vi "Get Size 1D.vi"(8 "error in (no error)":errorcluster, 11 "Abs_Array1D in":refnum<class "Abs_Array1D.lvclass">) -> (0 "error out":errorcluster, 2 "Size":i32, 3 "Abs_Array1D out":refnum<class "Abs_Array1D.lvclass">)   [LabVIEW 2021, in "Abs_Array1D.lvclass"]
uses:
  Abs_Array1D.lvclass
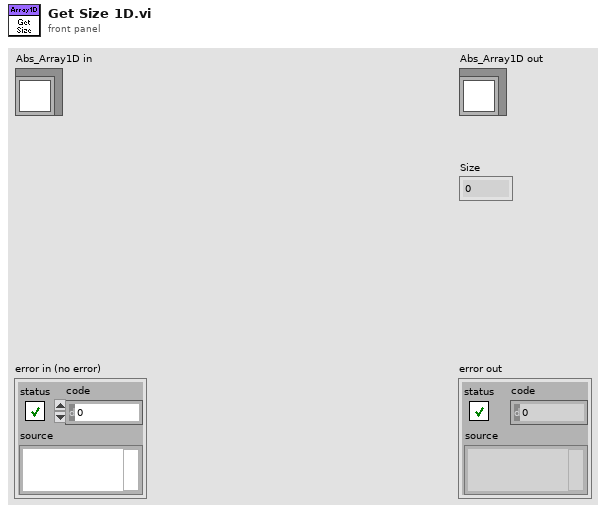
[diagram p1: front panel]
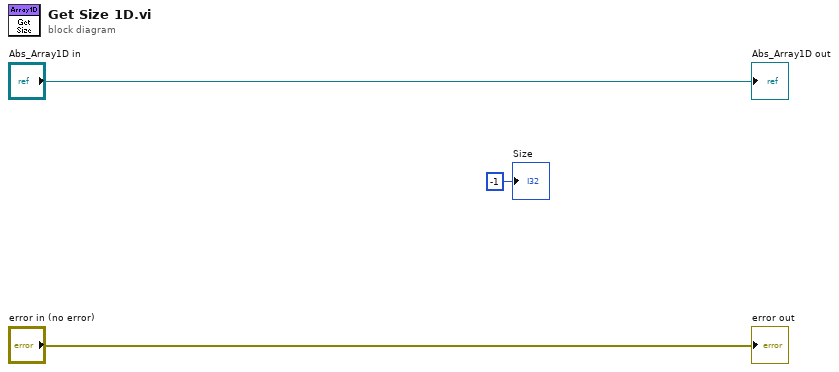
[diagram p0: block diagram]
diagram:
  "error out" <- "error in (no error)"
  "Abs_Array1D out" <- "Abs_Array1D in"
  "Size" <- -1 ("Size")
